vi "Decorate.vi"(10 "Event":refnum<class "Event.lvclass">, 11 "TEMPLATE Event in":refnum<class "TEMPLATE Event.lvclass">) -> (3 "TEMPLATE Event out":refnum<class "TEMPLATE Event.lvclass">)   [LabVIEW 2021, in "_Template.lvlib" / "Templates.lvlib" / "TEM Event.lvlib" / "TEMPLATE Event.lvclass"]
uses:
  TEMPLATE Event.lvclass
  <vilib>/Nathan Davis/jettl/jettl/Event/Event.lvclass
  TEMPLATE Event.lvclass/TEMPLATE Event.ctl
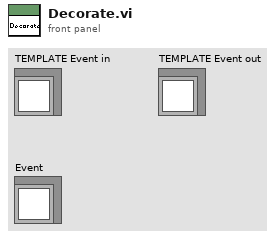
[diagram p1: front panel]
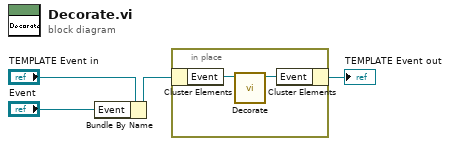
[diagram p0: block diagram]
diagram:
  n1 = Bundle By Name(cluster="TEMPLATE Event in", "Event"="Event") -> (w2:refnum<class "TEMPLATE Event.lvclass">)
  n2 = in-place {
    n3 = in-place-cluster #1(w2) -> ("Event"=w6:refnum<class "Event.lvclass">)
    n4 = call-dynamic "Decorate.vi"("Event in"=w6) -> ("Event out"=w5:refnum<class "Event.lvclass">)  [unwired: 10 in]
    n5 = in-place-cluster #1("Event"=w5) -> (→"TEMPLATE Event out":refnum<class "TEMPLATE Event.lvclass">)
  }
